vi "SearchNode.vi"(8 "error in (no error)":errorcluster, 10 "Node in":refnum<data-value>, 11 "SearchPriority in":refnum<class "SearchPriority.lvclass">) -> (0 "error out":errorcluster, 1 "found":bool, 2 "Node out":refnum<data-value>, 3 "SearchPriority out":refnum<class "SearchPriority.lvclass">)   [LabVIEW 2009, in "SearchPriority.lvclass"]
uses:
  SearchPriority.lvclass
  Node/Node.lvclass
  PriorityNode/PriorityNode.lvclass
  SearchPriority.lvclass/SearchPriority.ctl
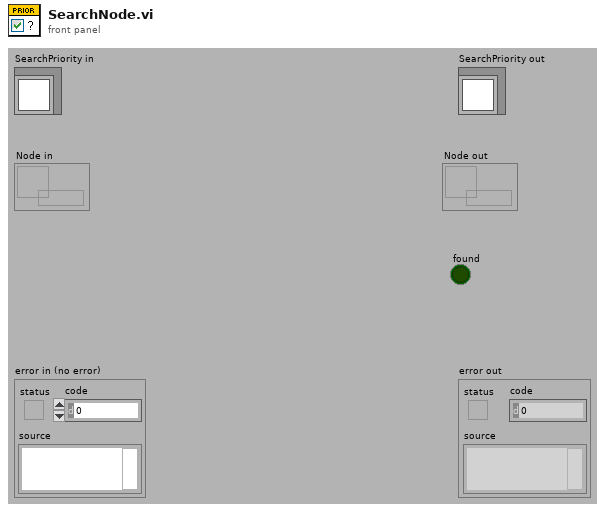
[diagram p1: front panel]
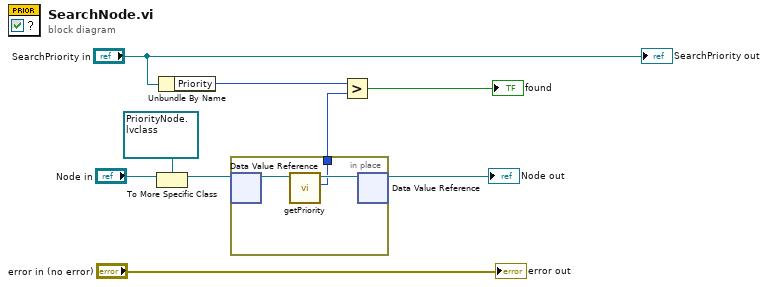
[diagram p0: block diagram]
diagram:
  n1 = To More Specific Class(target class=refnum<data-value> refnum ("data value reference"), reference="Node in") -> (specific class reference=w7:refnum<data-value>)  [unwired: 1 in, 1 out]
  n2 = Unbundle By Name("SearchPriority in") -> ("Priority"=w5:u8)
  n3 = in-place {
    in-place-border: [w10] -> w6
    n4 = in-place-dvr #1(w7) -> (w12:refnum<class "PriorityNode.lvclass">)  [unwired: 1 out]
    n5 = call "getPriority.vi"("PriorityNode in"=w12) -> ("Priority"=w10:u8, "PriorityNode out"=w11:refnum<class "PriorityNode.lvclass">)  [unwired: 8 in, 1 out]
    n6 = in-place-dvr #1(w11) -> (→"Node out":refnum<data-value>)  [unwired: 1 out]
  }
  n7 = Greater?(x=w5, y=w6) -> (0:→"found":bool)
  "error out" <- "error in (no error)"
  "SearchPriority out" <- "SearchPriority in"
